vi "Write Ver.vi"(8 "error in (no error)":errorcluster, 10 "Ver":u8=1, 11 "SMSD in":refnum<class "SMSD.lvclass">) -> (0 "error out":errorcluster, 3 "SMSD out":refnum<class "SMSD.lvclass">)   [LabVIEW 2021, in "SMSD.lvclass"]
uses:
  SMSD.lvclass
  SMSD.lvclass/SMSD.ctl
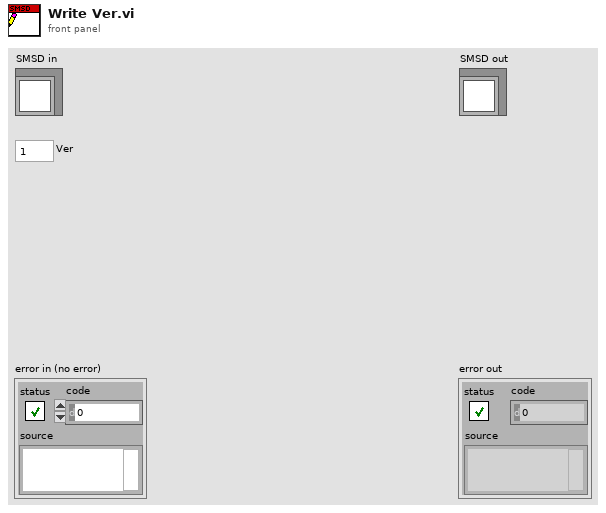
[diagram p1: front panel]
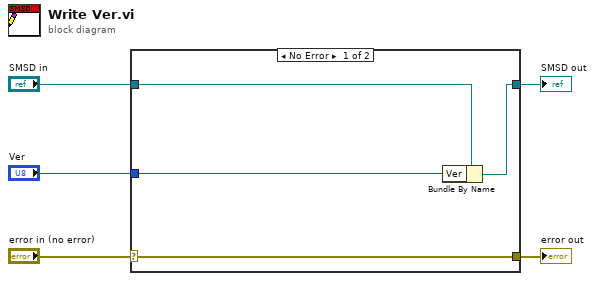
[diagram p0: block diagram]
diagram:
  n1 = case shown="No Error" "error in (no error)" {
    selector: "error in (no error)" -> [w9 w10]
    tunnel: [w9 w10] -> w4
    tunnel: [w7 w11] -> w2
    tunnel: "SMSD in" -> [w8 w11]
    tunnel: "Ver" -> [w6 _]
    frame No Error {
      n2 = Bundle By Name(cluster=w8, "Ver"=w6) -> (w7:refnum<class "SMSD.lvclass">)
    }
    frame Error {
    }
  }
  "error out" <- w4
  "SMSD out" <- w2
